vi "相机1影像dtXY-转换成机械手mm.vi"(11 "校准：相机1示教时影像坐标":T1 {"X" format="%#.3f"}) -> (0 "机械手移动量XY数组 mm":dbl[](array[numeric]), 2 "机械手移动量 mm":T1 {"X" format="%#.3f"})   [LabVIEW 2014]
uses:
  Controls/XYPos.ctl
  Global.vi
panel:
  out "机械手移动量 mm 2":T1 {"X" format="%#.3f"}
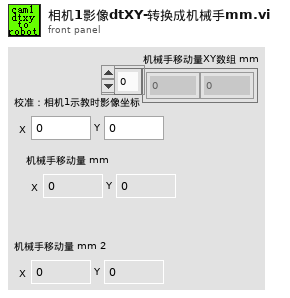
[diagram p1: front panel]
types:
  T1 = typedef "XYPos.ctl" = cluster{"X":dbl, "Y":dbl}
  T2 = typedef "OtherSpec.ctl" = cluster{"其它勾选类规格":T3, "其它数据类规格":T4, "相机名称":T5, "参数":cluster{"Mark1曝光时间":i32, "Mark2曝光时间":i32, "二维码曝光时间":i32}}
  T3 = typedef "其它勾选类规格.ctl" = cluster{"保存图片":bool, "上传设备状态数据":bool, "保存数据":bool, "开机默认开启监控摄像头":bool, "启用mark拍照 ":bool}
  T4 = typedef "其他数据类规格.ctl" = cluster{"相机1像素-毫米换算系数":dbl, "相机2像素-毫米换算系数":dbl, "D盘剩余空间预警(G)":dbl, "视频最长录制时间(秒)":dbl}
  T5 = typedef "相机名称品牌使用状态.ctl" = cluster{"相机1名称":T6, "相机2名称":T6, "Cam1启用":bool, "Cam2启用":bool, "Basler1":bool, "Basler2":bool}
  T6 = typedef "IMAQdx.ctl" = refnum<k21>
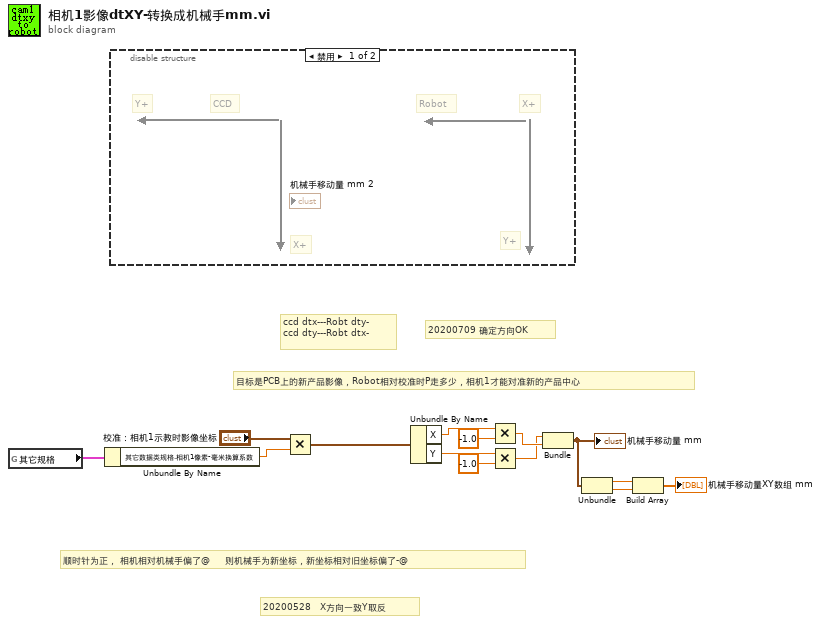
[diagram p0: block diagram]
diagram:
  # "20200709 确定方向OK"
  # "20200528   X方向一致Y取反"
  # "目标是PCB上的新产品影像，Robot相对校准时P走多少，相机1才能对准新的产品中心"
  # "顺时针为正， 相机相对机械手偏了@     则机械手为新坐标，新坐标相对旧坐标偏了-@"
  # "ccd dtx---Robt dty-\nccd dty---Robt dtx-"
  n1 = global read "Global.vi" "其它规格"() -> (w14:T2)
  n2 = Unbundle By Name(w14) -> ("其它数据类规格.相机1像素-毫米换算系数"=w12:dbl)
  n3 = disable-structure shown="禁用" {
    frame Disabled {
      # "CCD"
      # "Y+"
      # "X+"
      # "Y+"
      # "X+"
      # "Robot"
    }
    frame Enabled {
    }
  }
  n4 = Multiply(x="校准：相机1示教时影像坐标", y=w12) -> (x*y=w1:T1)
  n5 = Unbundle By Name(w1) -> ("X"=w11:dbl, "Y"=w10:dbl)
  n6 = Multiply(x=w11, y=-1.0) -> (x*y=w7:dbl)
  n7 = Multiply(x=w10, y=-1.0) -> (x*y=w6:dbl)
  n8 = Bundle(w6, w7) -> (w4:cluster{dbl, dbl})  [unwired: 1 in]
  "机械手移动量 mm" <- w4
  n9 = Unbundle(w4) -> (w5:dbl, w3:dbl)
  n10 = Build Array(w5, w3) -> (→"机械手移动量XY数组 mm":dbl[])
